vi "Closest Mass.vi"(11 "Data In":string) -> (3 "Data Out":string)   [LabVIEW 2018, in "Labview Python.lvlib"]
uses:
  Labview Python.lvlib
  Mass Analysis/Mass Analysis.lvlib
panel:
  in  "cluster":cluster{"Charge (e)":dbl[], "Mass (kg)":dbl[]}
  in  "output cluster":T1
  out "JSON string":string
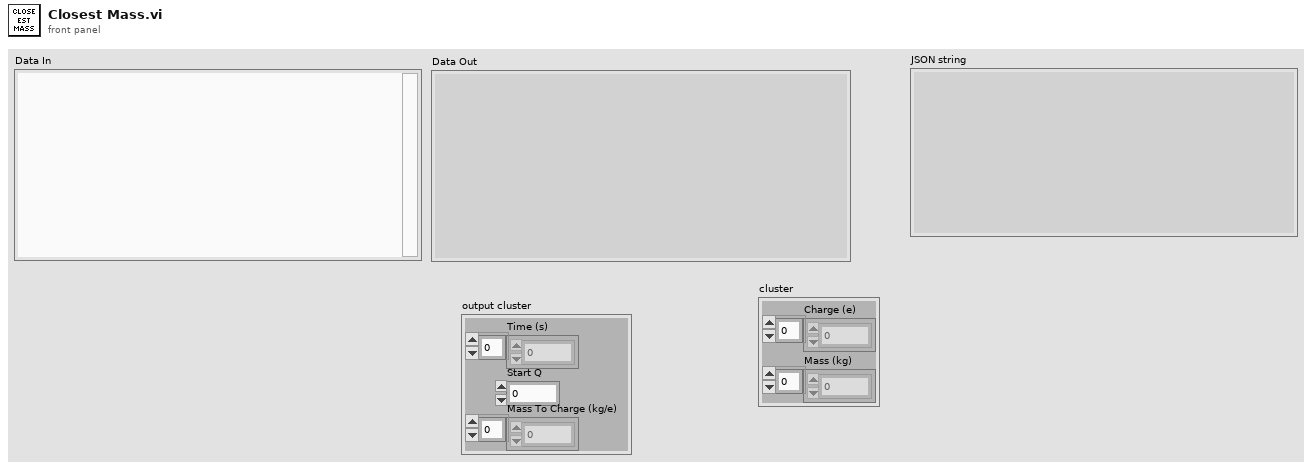
[diagram p1: front panel]
types:
  T1 = cluster{"Time (s)":dbl[], "Start Q":dbl, "Mass To Charge (kg/e)":dbl[]}
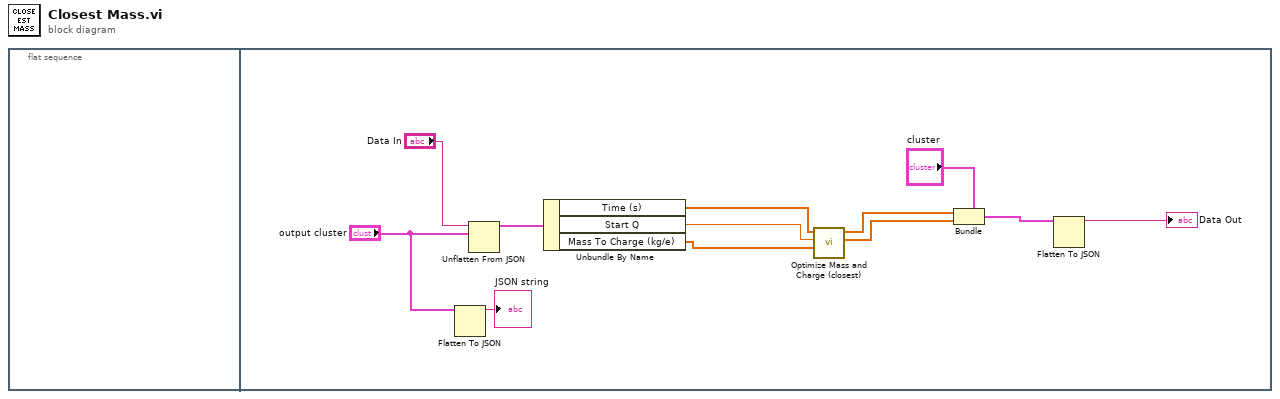
[diagram p0: block diagram]
diagram:
  n1 = flat-sequence {
    frame #0 {
    }
    frame #1 {
      n2 = Flatten To JSON(anything="output cluster") -> (JSON string=→"JSON string":string)  [unwired: 2 in, 1 out]
      n3 = Unflatten From JSON(JSON string="Data In", type and defaults="output cluster") -> (value=w11:T1)  [unwired: 5 in, 1 out]
      n4 = Unbundle By Name(w11) -> ("Time (s)"=w6:dbl[], "Start Q"=w5:dbl, "Mass To Charge (kg/e)"=w4:dbl[])
      n5 = call "Optimize Mass and Charge (closest).vi"("Mass/Q Subarray (kg/e)"=w4, "Start Q"=w5, "Time (s)"=w6) -> ("Mass"=w2:dbl[], "Q"=w3:dbl[])  [unwired: 5 in, 2 out]
      n6 = Bundle(cluster="cluster", "Charge (e)"=w3, "Mass (kg)"=w2) -> (w9:cluster{"Charge (e)":dbl[], "Mass (kg)":dbl[]})
      n7 = Flatten To JSON(anything=w9) -> (JSON string=→"Data Out":string)  [unwired: 2 in, 1 out]
    }
  }
